vi "MW_微波源设置.vi"() -> ()   [LabVIEW 2016]
uses:
  MW_ctl_Souce Freq..ctl
  MW_ctl_Powers.ctl
  MW_ctl_Power_single..ctl
  Microwave Source.lvlib
panel:
  in  "stop":bool
  out "Probe Current Freq(GHz)":dbl=nan format="%#.6p"
  out "LO Current Freq(GHz)":dbl=11.9 format="%#.6p"
  in  "MW Power":T1={"LO"={"Output"=TRUE, "Power dBm"=10.0}, "Probe"={"Output"=TRUE, "Power dBm"=-20.0}} {"LO"."Power dBm" format="%.3p"; "Probe"."Power dBm" format="%.3p"}
  in  "MW Source Freq.":T3={"start"=6000000000.0, "step"=1000000.0, "end"=8000000000.0, "iteration"=0.0, "diff"=50000000.0}
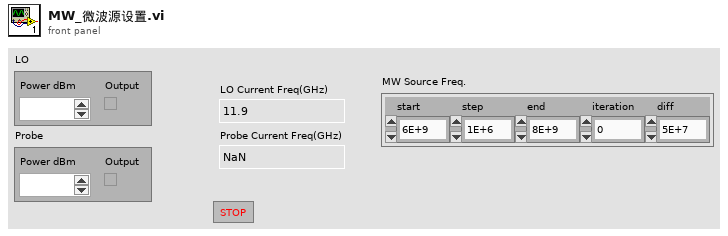
[diagram p1: front panel]
types:
  T1 = typedef "Microwave Source.lvlib/MW_ctl_Powers.ctl" = cluster{"LO":T2, "Probe":T2}
  T2 = typedef "Microwave Source.lvlib/MW_ctl_Power_single..ctl" = cluster{"Output":bool, "Power dBm":dbl}
  T3 = typedef "Microwave Source.lvlib/MW_ctl_Souce Freq..ctl" = cluster{"start":dbl, "step":dbl, "end":dbl, "iteration":dbl, "diff":dbl}
  T4 = typedef "Hardware_DeviceAddresses.ctl" = cluster{"ZI Device Name":string[][], "MW Source":T5, "Trigger Delayer VISA":refnum<visa-resource-name>}
  T5 = typedef "Microwave Source.lvlib/MW_ctl_DeviceHandles..ctl" = cluster{"LO VISA":refnum<visa-resource-name>, "Probe VISA":refnum<visa-resource-name>, "Qubits":refnum<visa-resource-name>[]}
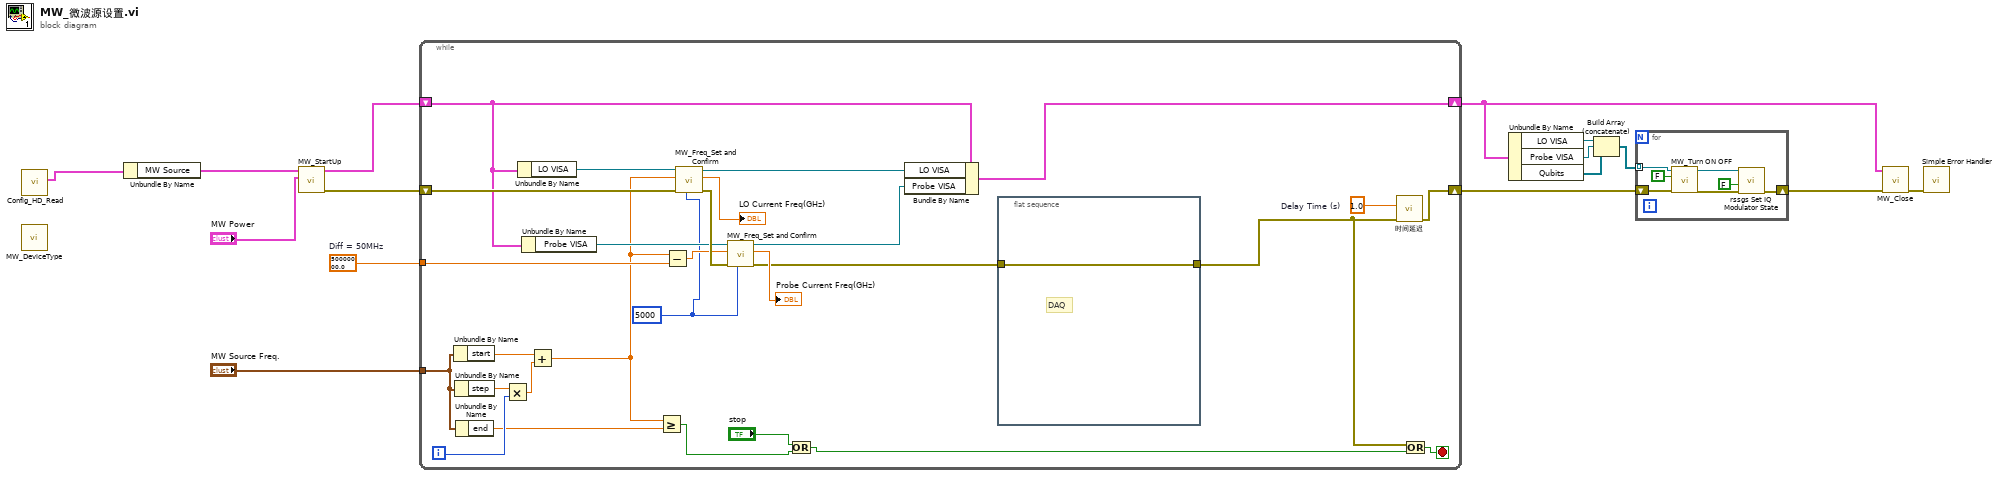
[diagram p0: block diagram]
diagram:
  w10 = 50000000.0  # Diff = 50MHz
  n1 = call "MW_DeviceType.vi"() -> ()  [unwired: 11 in, 1 out]
  n2 = call "Config_HD_Read.vi"() -> ("Dev Address"=w9:T4)  [unwired: 11 in]
  n3 = Unbundle By Name(w9) -> ("MW Source"=w8:T5)
  n4 = call "MW_StartUp.vi"("MW Power"="MW Power", "MW Source In"=w8) -> ("error out"=w12:errorcluster, "MW Source Out"=w11:T5)  [unwired: 8 in]
  n5 = while {
    tunnel: "MW Source Freq." -> [w23]
    tunnel: w10 -> [w31]
    shift-right: [w30] -> w6
    shift-left: w12 -> [w42]
    shift-right: [w26] -> w5
    shift-left: w11 -> [w29]
    i -> [w35]
    stop <- w21 stop-if-true
    w19 = 5000 ("Timout (500ms, -1=never)")
    w43 = 1.0  # Delay Time (s)
    n6 = Unbundle By Name(w23) -> ("start"=w37:dbl)
    n7 = Unbundle By Name(w23) -> ("step"=w38:dbl)
    n8 = Unbundle By Name(w23) -> ("end"=w22:dbl)
    n9 = Multiply(x=w38, y=w35) -> (x*y=w36:dbl)
    n10 = Unbundle By Name(w29) -> ("LO VISA"=w40:refnum<visa-resource-name>)
    n11 = Unbundle By Name(w29) -> ("Probe VISA"=w39:refnum<visa-resource-name>)
    n12 = Add(x=w37, y=w36) -> (x+y=w24:dbl)
    n13 = Greater Or Equal?(x=w24, y=w22) -> (x >= y?=w18:bool)
    n14 = Subtract(x=w24, y=w31) -> (x-y=w32:dbl)
    n15 = call "MW_Freq_Set and Confirm.vi"("Timout (5000ms, -1=never)"=w19, "错误输入（无错误）"=w42, "Set Frequency (Hz)"=w24, "VISA引用句柄输入"=w40) -> ("错误输出"=w41:errorcluster, "Current Freq(Hz)"=→"LO Current Freq(GHz)":dbl, "VISA引用句柄输出"=w28:refnum<visa-resource-name>)  [unwired: 5 in]
    n16 = call "MW_Freq_Set and Confirm.vi"("Timout (5000ms, -1=never)"=w19, "错误输入（无错误）"=w41, "Set Frequency (Hz)"=w32, "VISA引用句柄输入"=w39) -> ("错误输出"=w25:errorcluster, "Current Freq(Hz)"=→"Probe Current Freq(GHz)":dbl, "VISA引用句柄输出"=w27:refnum<visa-resource-name>)  [unwired: 5 in]
    n17 = Or(x="stop", y=w18) -> (x .or. y?=w17:bool)
    n18 = Bundle By Name(cluster=w29, "LO VISA"=w28, "Probe VISA"=w27) -> (w26:T5)
    n19 = flat-sequence {
      tunnel: [w44] -> w20
      tunnel: w25 -> [w44]
      frame #0 {
        # "DAQ"
      }
    }
    n20 = call "时间延迟"("error in (no error)"=w20, "Delay Time (s)"=w43) -> ("error out"=w30:errorcluster)  [unwired: 9 in]
    n21 = Or(x=w20, y=w17) -> (x .or. y?=w21:bool)
  }
  n22 = Unbundle By Name(w5) -> ("LO VISA"=w4:refnum<visa-resource-name>, "Probe VISA"=w3:refnum<visa-resource-name>, "Qubits"=w2:refnum<visa-resource-name>[])
  n23 = Build Array (concatenate)(w4, w3, w2) -> (w1:refnum<visa-resource-name>[])
  n24 = for {
    shift-right: [w46] -> w7
    shift-left: w6 -> [w51]
    tunnel: w1 -> [w49] mode=indexing
    n25 = call "MW_Turn ON OFF.vi"("错误输入（无错误）"=w51, "start MW source?"=FALSE, "VISA引用句柄输入"=w49) -> ("错误输出"=w47:errorcluster, "VISA引用句柄输出"=w48:refnum<visa-resource-name>)  [unwired: 7 in]
    n26 = call <instrlib>:"rssgs Set IQ Modulator State.vi"("error in (no error)"=w47, "IQ Modulator State (Off)"=FALSE, "VISA resource name"=w48) -> ("error out"=w46:errorcluster)  [unwired: 7 in, 1 out]
  }
  n27 = call "MW_Close.vi"("error in (no error)"=w7, "MW Source Out"=w5) -> ("error out"=w15:errorcluster)  [unwired: 9 in]
  n28 = call <vilib>:"Simple Error Handler.vi"("error in (no error)"=w15) -> ()  [unwired: 4 in, 5 out]
